vi "Clone VIs FG.vi"(7 "Action":T1, 8 "error in":errorcluster) -> (0 "error out":errorcluster, 3 "VIs":string[](array[string]))   [LabVIEW 2011]
uses:
  Clone VIs FG Enum.ctl
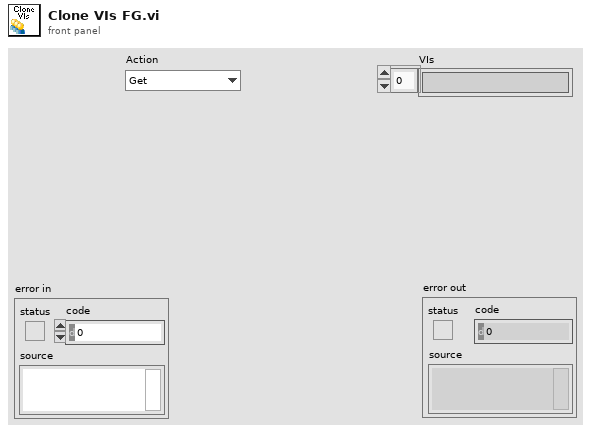
[diagram p1: front panel]
types:
  T1 = typedef "Clone VIs FG Enum.ctl" = enum16{"Get", "Get Active VIs", "Add Calling VI"}
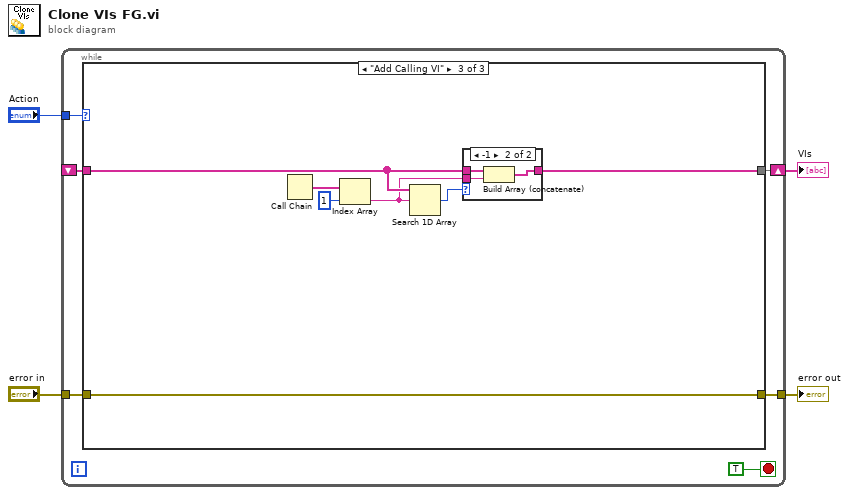
[diagram p0: block diagram]
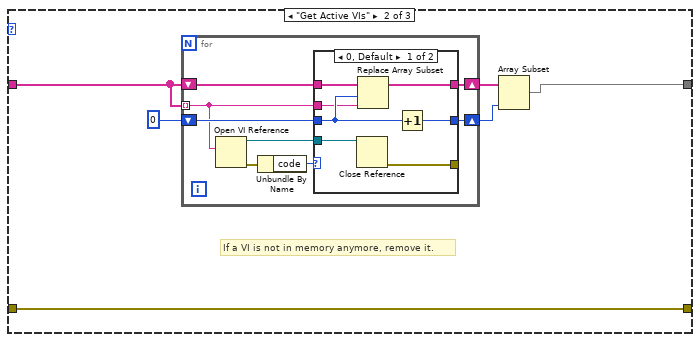
[diagram p3: hidden frame]
diagram:
  n1 = while {
    tunnel: "Action" -> [w9]
    shift-right: [w8] -> w1
    shift-left: _ -> [w7]
    tunnel: "error in" -> [w6]
    tunnel: [w5] -> w2
    stop <- TRUE stop-if-true
    n2 = case shown="\"Add Calling VI\"" w9 {
      tunnel: [w11 w13 w40] -> w8
      tunnel: w7 -> [w11 w14 w41]
      tunnel: w6 -> [w12 w18 w42]
      tunnel: [w12 w18 w42] -> w5
      frame "Get", Default {
      }
      frame "Get Active VIs" {
        # "If a VI is not in memory anymore, remove it."
        n3 = for {
          shift-right: [w22] -> w16
          shift-left: w14 -> [w23]
          tunnel: w14 -> [w19] mode=indexing
          shift-right: [w21] -> w15
          shift-left: 0 -> [w20]
          n4 = Open VI Reference(vi path=w19) -> (vi reference=w24:refnum<vi>, error out=w26:errorcluster)  [unwired: 5 in]
          n5 = Unbundle By Name(w26) -> ("code"=w25:i32)
          n6 = case shown="0, Default" w25 {
            tunnel: w24 -> [w33 _]
            tunnel: w23 -> [w32 w35]
            tunnel: [w29 w35] -> w22
            tunnel: [w30 w34] -> w21
            tunnel: w20 -> [w31 w34]
            tunnel: [w28 _] -> _
            tunnel: w19 -> [w27 _]
            frame 0, Default {
              n7 = Close Reference(reference=w33) -> (error out=w28:errorcluster)  [unwired: 1 in]
              n8 = Replace Array Subset(array=w32, new element=w27, index=w31) -> (w29:string[])
              n9 = Increment(x=w31) -> (x+1=w30:i32)
            }
            frame 1004 {
              # "VI not in memory"
            }
          }
        }
        n10 = Array Subset(array=w16, length=w15) -> (w13:string[])  [unwired: 1 in]
      }
      frame "Add Calling VI" {
        n11 = Call Chain() -> (call chain=w39:string[])
        n12 = Index Array(array=w39, index=1) -> (element=w37:string)
        n13 = Search 1D Array(1D array=w41, element=w37) -> (index of element=w36:i32)  [unwired: 1 in]
        n14 = case shown="-1" w36 {
          tunnel: w41 -> [w43 w46]
          tunnel: [w43 w45] -> w40
          tunnel: w37 -> [_ w44]
          frame 0, Default {
          }
          frame -1 {
            n15 = Build Array (concatenate)(w46, w44) -> (w45:string[])
          }
        }
      }
    }
  }
  "error out" <- w2
  "VIs" <- w1
